vi "Gyro_contraints.vi"(11 "angle":dbl) -> (3 "final angle":dbl)   [LabVIEW 2014]
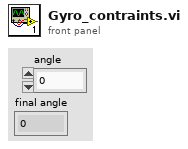
[diagram p1: front panel]
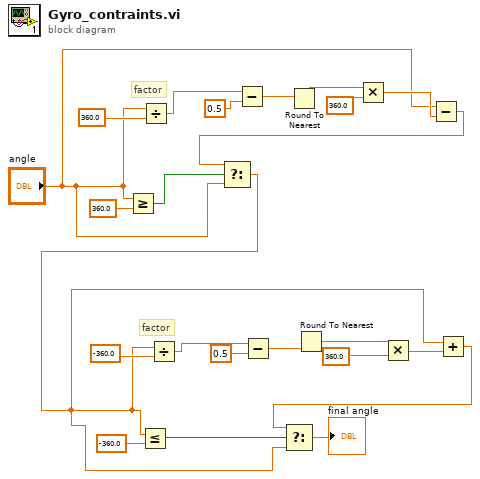
[diagram p0: block diagram]
diagram:
  # "factor"
  # "factor"
  n1 = Greater Or Equal?(x="angle", y=360.0) -> (x >= y?=w22:bool)
  n2 = Divide(x="angle", y=360.0) -> (x/y=w20:dbl)
  n3 = Subtract(x=w20, y=0.5) -> (x-y=w18:dbl)
  n4 = Round To Nearest(number=w18) -> (nearest integer value=w17:dbl)
  n5 = Multiply(x=w17, y=360.0) -> (x*y=w15:dbl)
  n6 = Subtract(x="angle", y=w15) -> (x-y=w14:dbl)
  n7 = Select(t=w14, s=w22, f="angle") -> (s? t:f=w3:dbl)
  n8 = Less Or Equal?(x=w3, y=-360.0) -> (x <= y?=w12:bool)
  n9 = Divide(x=w3, y=-360.0) -> (x/y=w10:dbl)
  n10 = Subtract(x=w10, y=0.5) -> (x-y=w8:dbl)
  n11 = Round To Nearest(number=w8) -> (nearest integer value=w7:dbl)
  n12 = Multiply(x=w7, y=360.0) -> (x*y=w1:dbl)
  n13 = Add(x=w3, y=w1) -> (x+y=w5:dbl)
  n14 = Select(t=w5, s=w12, f=w3) -> (s? t:f=→"final angle":dbl)
